vi "Demo Variables.vi"() -> ()   [LabVIEW 2021, in "HttpServer.lvlib"]
uses:
  HttpServer.lvlib
panel:
  out "Variables out":map{string, string[]}(c390)
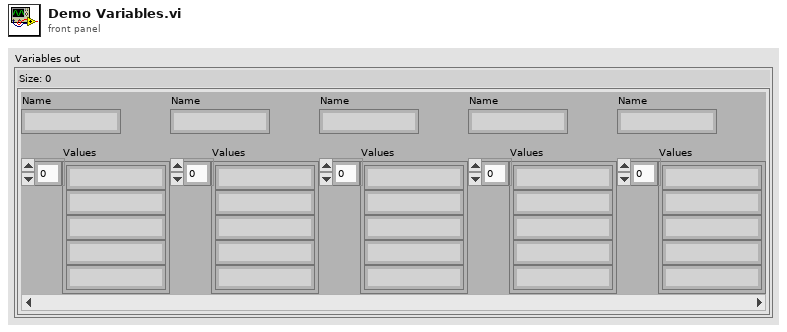
[diagram p1: front panel]
types:
  T1 = cluster{"status":bool, "code":i32, "source":string, "DBL":dbl}
  T2 = cluster{"data":string, "method":string, "path":string, "query":string, "url":string}
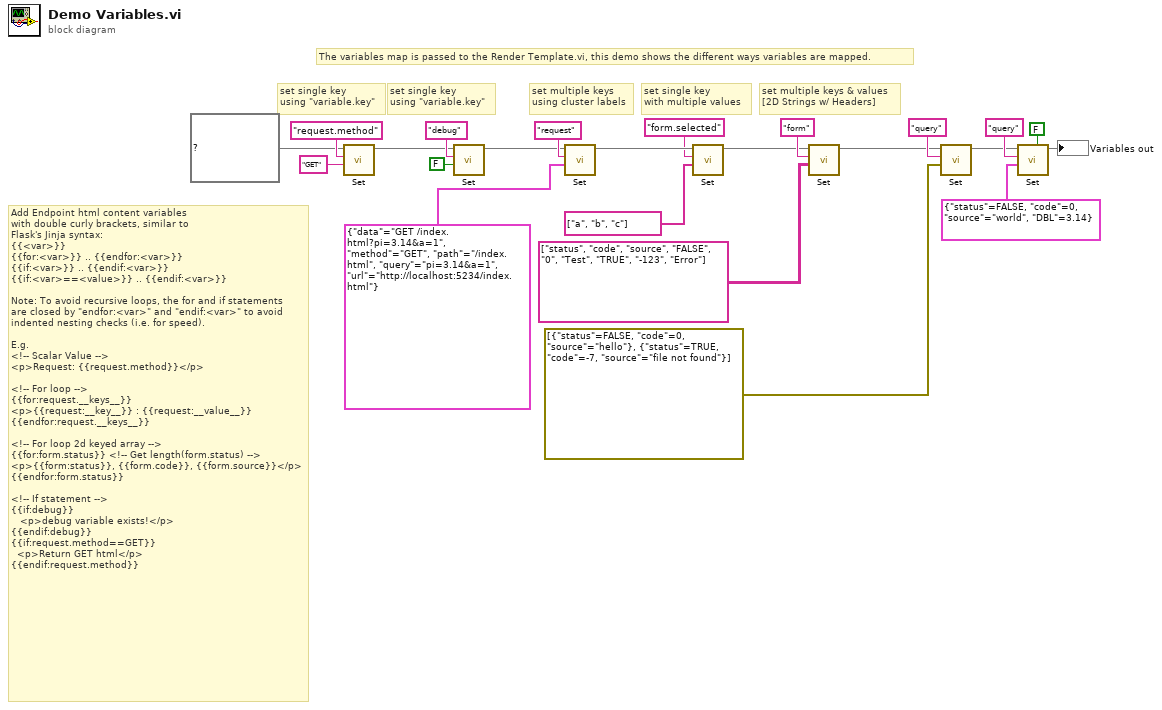
[diagram p0: block diagram]
diagram:
  # "Add Endpoint html content variables \nwith double curly brackets, similar to\nFlask's Jinja syntax:\n{{<var>}}\n{{for:<var>}} .. {{endfor:<var>}}\n{{if:<var>}} .. {{endif:<var>}}\n{{if:<var>==<value>}} .. {{endif:<var>}}\n\nNote: To avoid recursive loops, the for and if statements\nare closed by \"endfor:<var>\" and \"endif:<var>\" to avoid\nindented nesting checks (i.e. for speed).\n\nE.g.\n<!-- Scalar Value -->\n<p>Request: {{request.method}}</p>\n\n<!-- For loop -->\n{{for:request.__keys__}}\n<p>{{request:__key__}} : {{request:__value__}}\n{{endfor:request.__keys__}}\n\n<!-- For loop 2d keyed array -->\n{{for:form.status}} <!-- Get length(form.status) -->\n<p>{{form:status}}, {{form.code}}, {{form.source}}</p>\n{{endfor:form.status}}\n\n<!-- If statement -->\n{{if:debug}}\n   <p>debug variable exists!</p>\n{{endif:debug}}\n{{if:request.method==GET}}\n  <p>Return GET html</p>\n{{endif:request.method}}"
  # "The variables map is passed to the Render Template.vi, this demo shows the different ways variables are mapped."
  # "set single key\nusing \"variable.key\""
  # "set multiple keys & values\n[2D Strings w/ Headers]"
  # "set single key\nwith multiple values"
  # "set multiple keys\nusing cluster labels"
  # "set single key\nusing \"variable.key\""
  n1 = call "Set.vi"("Value [Scalar, Cluster, 1D_Clusters, 2D_String]"="GET" ("key"), "Name"="request.method" ("key"), "Variables in"=map{string, string[]} {} ("Keys")) -> ("Variables out"=w5:map{string, string[]})  [unwired: 7 in, 1 out]
  n2 = call "Set.vi"("Value [Scalar, Cluster, 1D_Clusters, 2D_String]"=FALSE, "Name"="debug" ("key"), "Variables in"=w5) -> ("Variables out"=w4:map{string, string[]})  [unwired: 7 in, 1 out]
  n3 = call "Set.vi"("Value [Scalar, Cluster, 1D_Clusters, 2D_String]"=T2 {"data"="GET /index.html?pi=3.14&a=1", "method"="GET", "path"="/index.html", "query"="pi=3.14&a=1", "url"="http://localhost:5234/index.html"} ("request"), "Name"="request" ("key"), "Variables in"=w4) -> ("Variables out"=w19:map{string, string[]})  [unwired: 7 in, 1 out]
  n4 = call "Set.vi"("Value [Scalar, Cluster, 1D_Clusters, 2D_String]"=string[] ["a", "b", "c"], "Name"="form.selected" ("Variable[.Key]"), "Variables in"=w19) -> ("Variables out"=w15:map{string, string[]})  [unwired: 7 in, 1 out]
  n5 = call "Set.vi"("Value [Scalar, Cluster, 1D_Clusters, 2D_String]"=string[][] [["status", "code", "source"], ["FALSE", "0", "Test"], ["TRUE", "-123", "Error"]], "Name"="form" ("Variable[.Key]"), "Variables in"=w15) -> ("Variables out"=w12:map{string, string[]})  [unwired: 7 in, 1 out]
  n6 = call "Set.vi"("Value [Scalar, Cluster, 1D_Clusters, 2D_String]"=errorcluster[] [{"status"=FALSE, "code"=0, "source"="hello"}, {"status"=TRUE, "code"=-7, "source"="file not found"}], "Name"="query" ("Variable[.Key]"), "Variables in"=w12) -> ("Variables out"=w9:map{string, string[]})  [unwired: 7 in, 1 out]
  n7 = call "Set.vi"("Append Key? (F=Replace)"=FALSE, "Value [Scalar, Cluster, 1D_Clusters, 2D_String]"=T1 {"status"=FALSE, "code"=0, "source"="world", "DBL"=3.14} ("error constant"), "Name"="query" ("Variable[.Key]"), "Variables in"=w9) -> ("Variables out"=→"Variables out":map{string, string[]})  [unwired: 6 in, 1 out]
